vi "Remove Column.vi"(8 "error in (no error)":errorcluster, 11 "DataGrid Config Dialog in":refnum<class "DataGrid Config Dialog.lvclass">) -> (0 "error out":errorcluster, 3 "DataGrid Config Dialog out":refnum<class "DataGrid Config Dialog.lvclass">)   [LabVIEW 2018, in "DataGrid Config Dialog.lvclass"]
uses:
  DataGrid Config Dialog.lvclass
  DataGrid Config Dialog.lvclass/DataGrid Config Dialog.ctl
  DataGrid Config/Edit Configuration Actions.ctl
  DataGrid Config/DataGrid Config.lvclass
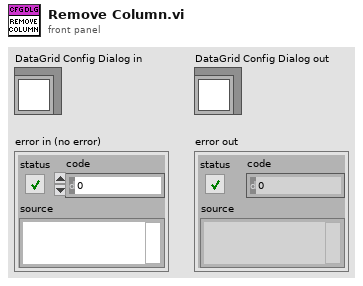
[diagram p1: front panel]
types:
  T1 = typedef "DataGrid Config.lvclass/Edit Configuration Actions.ctl" = enum16{"Add", "Remove", "Update", "Move Up", "Move Down"}
  T2 = enum8{"Enabled", "Disabled", "Disabled and Grayed Out"}
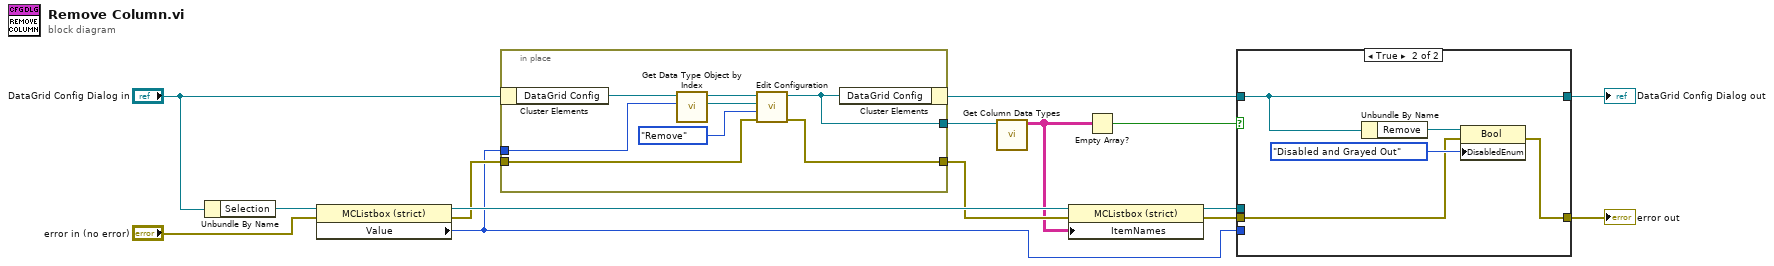
[diagram p0: block diagram]
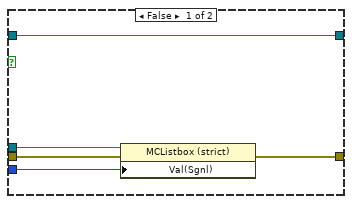
[diagram p2: hidden frame]
diagram:
  n1 = Unbundle By Name("DataGrid Config Dialog in") -> ("Selection"=w8:refnum<vi>)
  n2 = property class="MCListbox (strict)"(reference=w8, error in="error in (no error)") -> (reference out=w7:refnum<vi>, error out=w6:errorcluster, "Value"=w3:i32)
  n3 = in-place {
    in-place-border: w3 -> [w22]
    in-place-border: [w18] -> w5
    in-place-border: w6 -> [w17]
    in-place-border: [w16] -> w4
    n4 = in-place-cluster #1("DataGrid Config Dialog in") -> ("DataGrid Config"=w23:refnum<class "DataGrid Config.lvclass">)
    n5 = call "Get Data Type Object by Index.vi"("Index"=w22, "DataGrid Config in"=w23) -> ("Data Type Object"=w20:refnum<class "Generic Data Type.lvclass">, "DataGrid Config (dup)"=w21:refnum<class "DataGrid Config.lvclass">)  [unwired: 7 in, 1 out]
    n6 = call "Edit Configuration.vi"("error in (no error)"=w17, "Edit Configuration Actions"=Edit_Configuration_Actions."Remove", "Data Type Object"=w20, "DataGrid Config in"=w21) -> ("error out"=w16:errorcluster, "DataGrid Config out"=w18:refnum<class "DataGrid Config.lvclass">)  [unwired: 6 in]
    n7 = in-place-cluster #1("DataGrid Config"=w18) -> (w13:refnum<class "DataGrid Config Dialog.lvclass">)
  }
  n8 = call "Get Column Data Types.vi"("DataGrid Config"=w5) -> ("Column Data Type Names"=w2:string[][])  [unwired: 10 in]
  n9 = property class="MCListbox (strict)"(reference=w7, error in=w4, "ItemNames"=w2) -> (reference out=w9:refnum<vi>, error out=w11:errorcluster)
  n10 = Empty Array?(array=w2) -> (empty?=w1:bool)
  n11 = case shown="True" w1 {
    tunnel: w13 -> [w28 w33]
    tunnel: [w28 w33] -> w12
    tunnel: w11 -> [w26 w30]
    tunnel: [w25 w29] -> w10
    tunnel: w9 -> [w27 _]
    tunnel: w3 -> [w24 _]
    frame False {
      n12 = property class="MCListbox (strict)"(reference=w27, error in=w26, "Val(Sgnl)"=w24) -> (error out=w25:errorcluster)  [unwired: 1 out]
    }
    frame True {
      n13 = Unbundle By Name(w33) -> ("Remove"=w32:refnum<vi>)
      n14 = property class="Bool"(reference=w32, error in=w30, "DisabledEnum"=T2."Disabled and Grayed Out" ("Disabled")) -> (error out=w29:errorcluster)  [unwired: 1 out]
    }
  }
  "DataGrid Config Dialog out" <- w12
  "error out" <- w10
